vi "Programacion parcial 2 5.vi"() -> ()   [LabVIEW 2011]
uses:
  Control arreglo.ctl
panel:
  out "Array 2":bool[](array[boolean])
  out "Array":i32[](array[slide]) scale=0.0..60.0
  # "Encender un led cuando la temperatura sbrepase 60"
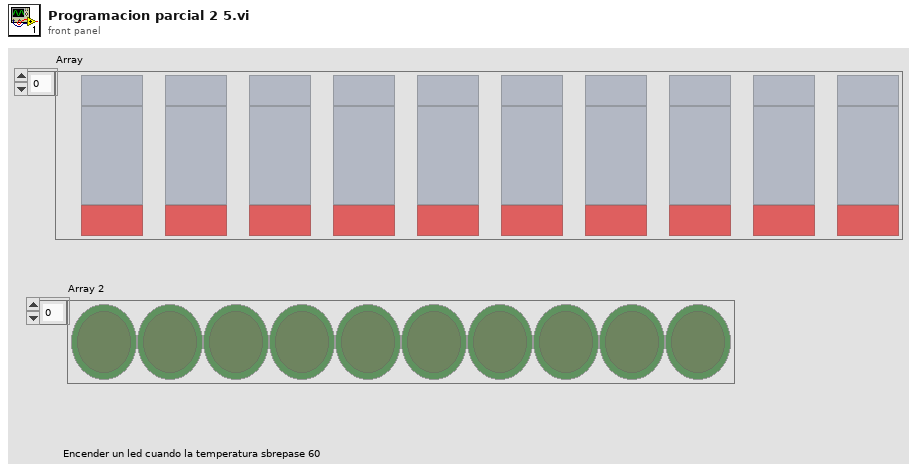
[diagram p1: front panel]
types:
  T1 = typedef "Control arreglo.ctl" = enum16{"Inicializar", "Rellenar temperatura", "Encender led", "Final"}
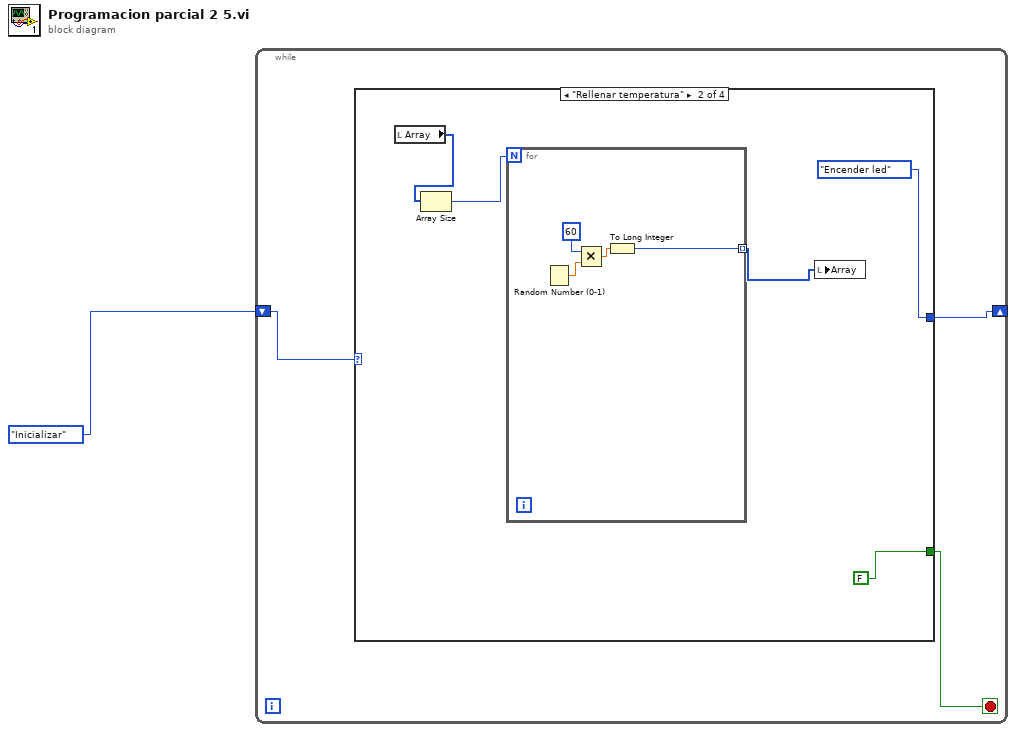
[diagram p0: block diagram]
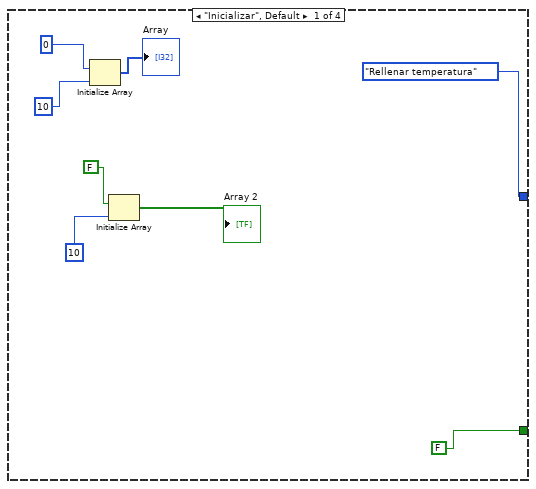
[diagram p2: hidden frame]
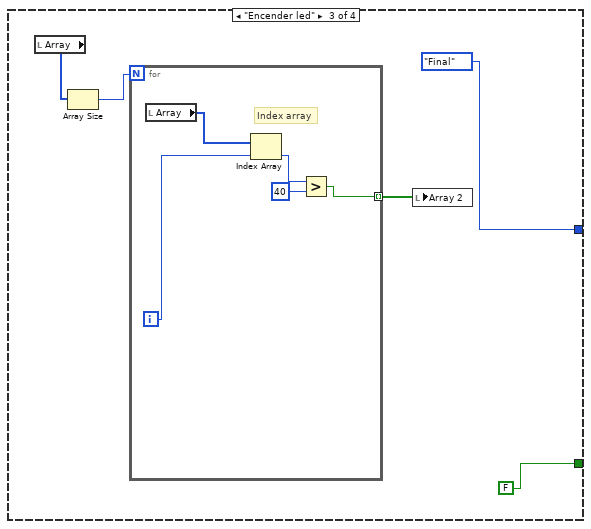
[diagram p3: hidden frame]
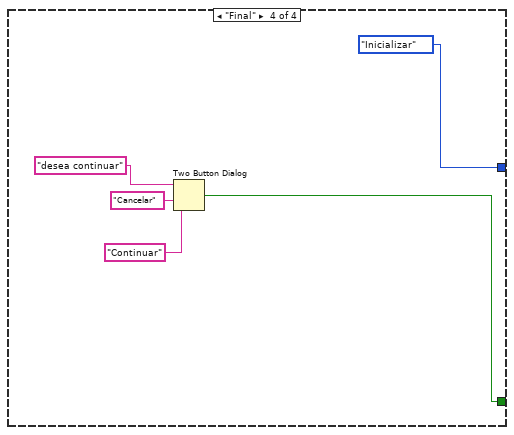
[diagram p4: hidden frame]
diagram:
  n1 = while {
    shift-right: [w3] -> _
    shift-left: Control_arreglo."Inicializar" -> [w4]
    stop <- w2 stop-if-true
    n2 = case shown="\"Rellenar temperatura\"" w4 {
      tunnel: [Control_arreglo."Rellenar temperatura" Control_arreglo."Encender led" Control_arreglo."Final" Control_arreglo."Inicializar"] -> w3
      tunnel: [FALSE FALSE FALSE w32] -> w2
      frame "Inicializar", Default {
        n3 = Initialize Array(0, 10) -> (→"Array":i32[])
        n4 = Initialize Array(FALSE, 10) -> (→"Array 2":bool[])
      }
      frame "Rellenar temperatura" {
        n5 = local read "Array"() -> (w17:i32[])
        n6 = Array Size(array=w17) -> (size(s)=w16:i32)
        n7 = for {
          N: w16 -> [_]
          tunnel: [w21] -> w15 mode=indexing
          n8 = Random Number (0-1)() -> (number: 0 to 1=w19:dbl)
          n9 = Multiply(x=60, y=w19) -> (x*y=w18:dbl)
          n10 = To Long Integer(number=w18) -> (32bit integer=w21:i32)
        }
        n11 = local write "Array"(w15) -> ()
      }
      frame "Encender led" {
        n12 = local read "Array"() -> (w26:i32[])
        n13 = Array Size(array=w26) -> (size(s)=w25:i32)
        n14 = for {
          N: w25 -> [_]
          tunnel: [w27] -> w24 mode=indexing
          i -> [w30]
          # "Index array"
          n15 = local read "Array"() -> (w31:i32[])
          n16 = Index Array(array=w31, index=w30) -> (element=w29:i32)
          n17 = Greater?(x=w29, y=40) -> (0:w27:bool)
        }
        n18 = local write "Array 2"(w24) -> ()
      }
      frame "Final" {
        n19 = Two Button Dialog(message="desea continuar", 1:"Continuar" ("F button name (\"Cancel\")"), 2:"Cancelar" ("T button name (\"OK\")")) -> (T button?=w32:bool)
      }
    }
  }
